vi "Movil SubVI.vi"(7 "Reset":bool, 8 "error in (no error)":errorcluster, 9 "Motor Izquierda":dbl(slide) scale=-100.0..100.0, 10 "Motor Derecha":dbl(slide) scale=-100.0..100.0, 11 "Ref Plano":refnum<vi>) -> (0 "error out":errorcluster, 1 "Distancia":dbl, 2 "Angulo":dbl, 3 "Plano de trabajo":picture, 5 "Button Down":bool)   [LabVIEW 2017]
uses:
  <vilib>/picture/picture.llb/imagedata.ctl
panel:
  out "new picture":picture
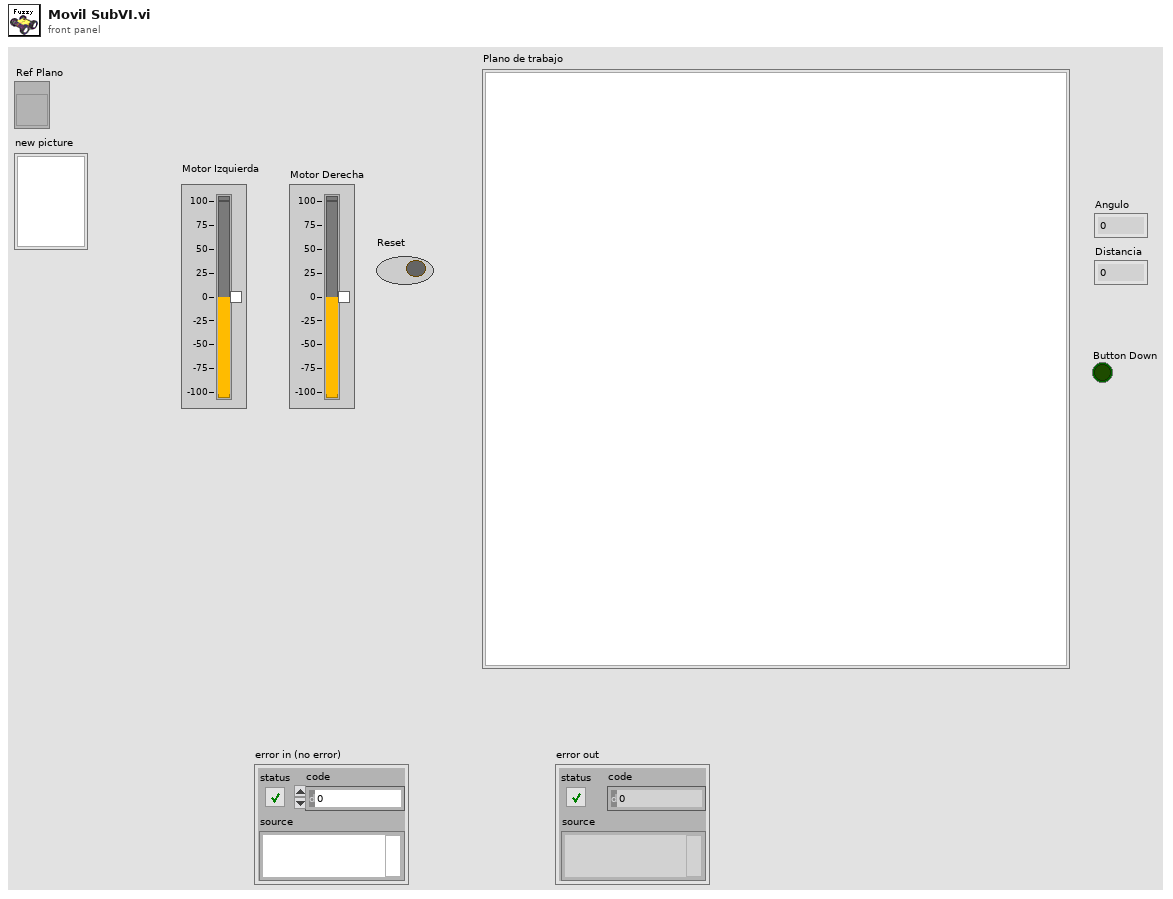
[diagram p1: front panel]
types:
  T1 = typedef "imagedata.ctl" = cluster{"image type":i32, "image depth":i32, "image":u8[], "mask":u8[], "colors":u32[], "Rectangle":cluster{"left":i16, "top":i16, "right":i16, "bottom":i16}}
  T2 = typedef "LVMouseTypeDef.ctl" = cluster{"Mouse Position":cluster{"X":i32, "Y":i32}, "Mouse Modifiers":cluster{"Button Down":bool, "Shift Mod":bool, "Menu Mod":bool, "Option Mod":bool}}
  T3 = cluster{"Button Down":bool, "Shift Mod":bool, "Menu Mod":bool, "Option Mod":bool}
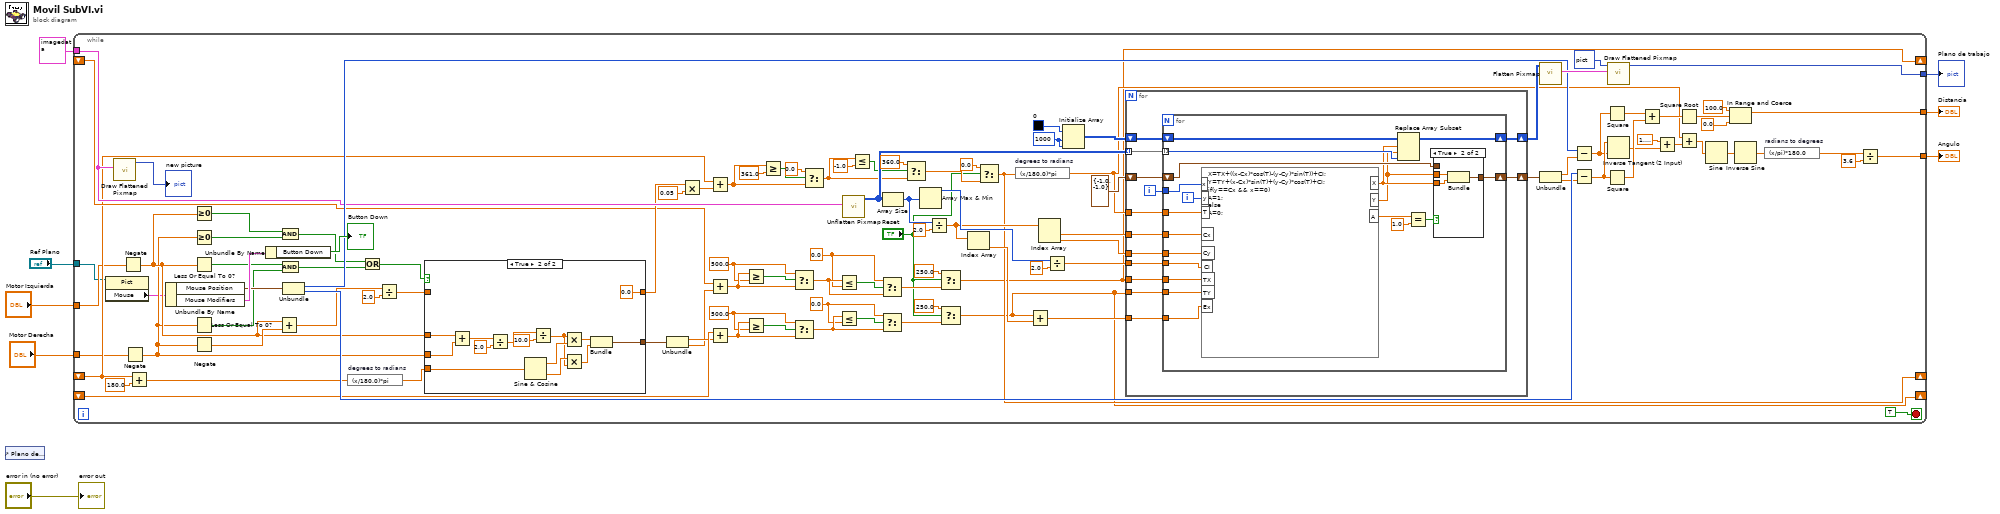
[diagram p0: block diagram]
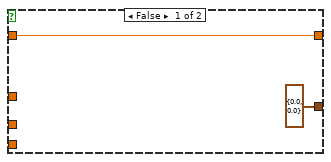
[diagram p2: hidden frame]
diagram:
  n1 = control-ref of="Plano de trabajo"() -> ()  [unwired: 1 out]
  n2 = while {
    shift-right: [w64] -> _
    shift-left: _ -> [w27]
    tunnel: T1 {"image type"=0, "image depth"=24, "image"=array[11970 elements], "mask"=[], "colors"=[], "Rectangle"={"left"=0, "top"=0, "right"=57, "bottom"=70}} ("image data") -> [w65]
    shift-right: [w24] -> _
    shift-left: _ -> [w38]
    shift-right: [w23] -> _
    shift-left: _ -> [w37]
    tunnel: "Motor Izquierda" -> [w17]
    tunnel: "Motor Derecha" -> [w16]
    tunnel: [w15] -> w5
    tunnel: [w14] -> w4
    tunnel: "Ref Plano" -> [w10]
    tunnel: [w9] -> w3
    stop <- TRUE stop-if-true
    w32 = 0.0 ("y")
    w34 = 500.0 ("y")
    w33 = 0.0 ("y")
    w35 = 500.0 ("y")
    w105 = 1000 ("dimension size")
    n3 = property class="Pict"(reference=w10) -> ("Mouse"=w11:T2)  [unwired: 1 in, 2 out]
    n4 = call <vilib>:"Draw Flattened Pixmap.vi"("image data"=w65) -> ("new picture"=→"new picture":picture)  [unwired: 8 in]
    n5 = Negate(x=w17) -> (-x=w13:dbl)
    n6 = Negate(x=w16) -> (-x=w12:dbl)
    n7 = Add(x=w27, y=180.0) -> (x+y=w25:dbl)
    n8 = Unbundle By Name(w11) -> ("Mouse Position"=w94:cluster{"X":i32, "Y":i32}, "Mouse Modifiers"=w104:T3)
    n9 = Greater Or Equal To 0?(x=w13) -> (x >= 0?=w59:bool)
    n10 = Greater Or Equal To 0?(x=w12) -> (x >= 0?=w58:bool)
    n11 = Less Or Equal To 0?(x=w13) -> (x <= 0?=w57:bool)
    n12 = Less Or Equal To 0?(x=w12) -> (x <= 0?=w56:bool)
    n13 = Negate(x=w12) -> (-x=w62:dbl)
    n14 = Unbundle By Name(w104) -> ("Button Down"=→"Button Down":bool)
    n15 = Add(x=w13, y=w62) -> (x+y=w61:dbl)
    n16 = And(x=w59, y=w58) -> (x .and. y?=w55:bool)
    n17 = And(x=w57, y=w56) -> (x .and. y?=w54:bool)
    n18 = Unbundle(w94) -> ("X"=w88:i32, "Y"=w90:i32)
    n19 = expression code="(x/180.0)*pi" "degrees to radians"(w25) -> (w31:dbl)
    n20 = Or(x=w55, y=w54) -> (x .or. y?=w53:bool)
    n21 = Divide(x=w61, y=2.0) -> (x/y=w52:dbl)
    n22 = case shown="True" w53 {
      tunnel: w52 -> [w118 _]
      tunnel: [w118 0.0] -> w51
      tunnel: w13 -> [_ w131]
      tunnel: w12 -> [_ w130]
      tunnel: w31 -> [_ w125]
      tunnel: [cluster{dbl, dbl} {0.0, 0.0} w119] -> w30
      frame False {
      }
      frame True {
        n23 = Add(x=w131, y=w130) -> (x+y=w129:dbl)
        n24 = Divide(x=w129, y=2.0) -> (x/y=w127:dbl)
        n25 = Sine & Cosine(0:w125) -> (1:w123:dbl, 2:w124:dbl)
        n26 = Divide(x=w127, y=10.0) -> (x/y=w122:dbl)
        n27 = Multiply(x=w122, y=w123) -> (x*y=w121:dbl)
        n28 = Multiply(x=w124, y=w122) -> (x*y=w120:dbl)
        n29 = Bundle(w121, w120) -> (w119:cluster{dbl, dbl})  [unwired: 1 in]
      }
    }
    n30 = Unbundle(w30) -> (w29:dbl, w28:dbl)
    n31 = Multiply(x=w51, y=0.05) -> (x*y=w69:dbl)
    n32 = Add(x=w27, y=w69) -> (x+y=w73:dbl)
    n33 = Add(x=w37, y=w28) -> (x+y=w43:dbl)
    n34 = Add(x=w38, y=w29) -> (x+y=w46:dbl)
    n35 = Greater Or Equal?(x=w43, y=w34) -> (x >= y?=w44:bool)
    n36 = Greater Or Equal?(x=w46, y=w35) -> (x >= y?=w45:bool)
    n37 = Greater Or Equal?(x=w73, y=361.0) -> (x >= y?=w75:bool)
    n38 = Select(t=w34, s=w44, f=w43) -> (s? t:f=w39:dbl)
    n39 = Select(t=w35, s=w45, f=w46) -> (s? t:f=w50:dbl)
    n40 = Select(t=0.0, s=w75, f=w73) -> (s? t:f=w66:dbl)
    n41 = Less Or Equal?(x=w39, y=w32) -> (x <= y?=w42:bool)
    n42 = Less Or Equal?(x=w50, y=w33) -> (x <= y?=w47:bool)
    n43 = call <vilib>:"Unflatten Pixmap.vi"("image data"=w65) -> ("24-bit pixmap"=w115:u32[][])  [unwired: 4 in, 6 out]
    n44 = Less Or Equal?(x=w66, y=-1.0) -> (x <= y?=w71:bool)
    n45 = Select(t=w32, s=w42, f=w39) -> (s? t:f=w40:dbl)
    n46 = Select(t=w33, s=w47, f=w50) -> (s? t:f=w49:dbl)
    n47 = Array Size(array=w115) -> (size(s)=w111:i32[])
    n48 = Select(t=360.0, s=w71, f=w66) -> (s? t:f=w67:dbl)
    n49 = Array Max & Min(array=w111) -> (max value=w109:i32)  [unwired: 3 out]
    n50 = Divide(x=w111, y=2.0) -> (x/y=w102:dbl[])
    n51 = Select(t=250.0, s="Reset", f=w40) -> (s? t:f=w23:dbl)
    n52 = Select(t=250.0, s="Reset", f=w49) -> (s? t:f=w24:dbl)
    n53 = Index Array(array=w102) -> (element=w101:dbl)  [unwired: 1 in]
    n54 = Select(t=0.0, s="Reset", f=w67) -> (s? t:f=w64:dbl)
    n55 = expression code="(x/180.0)*pi" "degrees to radians"(w64) -> (w82:dbl)
    n56 = Add(x=w24, y=w101) -> (x+y=w97:dbl)
    n57 = Index Array(array=w102) -> (element #1=w100:dbl, element #2=w99:dbl)  [unwired: 2 in]
    n58 = Divide(x=w109, y=2.0) -> (x/y=w98:dbl)
    n59 = Initialize Array(u32 0, w105, w105) -> (w108:u32[][])
    n60 = for {
      shift-right: [w141] -> w114
      shift-left: w108 -> [w145]
      tunnel: w82 -> [w143]
      tunnel: w115 -> [w142] mode=indexing
      tunnel: w100 -> [w140]
      tunnel: w99 -> [w139]
      tunnel: w98 -> [w138]
      tunnel: w23 -> [w137]
      tunnel: w24 -> [w136]
      tunnel: w97 -> [w135]
      shift-right: [w133] -> w95
      shift-left: cluster{dbl, dbl} {-1.0, -1.0} -> [w134]
      i -> [w144]
      n61 = for {
        shift-right: [w161] -> w141
        shift-left: w145 -> [w163]
        tunnel: w144 -> [w153]
        tunnel: w143 -> [w164]
        tunnel: w142 -> [w162] mode=indexing
        tunnel: w140 -> [w160]
        tunnel: w139 -> [w159]
        tunnel: w138 -> [w158]
        tunnel: w137 -> [w150]
        tunnel: w136 -> [w152]
        tunnel: w135 -> [w149]
        shift-right: [w154] -> w133
        shift-left: w134 -> [w157]
        i -> [w151]
        n62 = formula code="X=TX+((x-Cx)*cos(T)-(y-Cy)*sin(T))+CI;\nY=TY+(x-Cx)*sin(T)+(y-Cy)*cos(T)+CI;\nif(y==Cx && x==0)\nA=1;\nelse\nA=0;"("x"=w153, "y"=w151, "T"=w164, "Cx"=w160, "Cy"=w159, "CI"=w158, "TX"=w150, "TY"=w152, "Ex"=w149) -> ("X"=w156:dbl, "Y"=w155:dbl, "A"=w148:dbl)
        n63 = Replace Array Subset(array=w163, new element=w162, index (row)=w156, index (col)=w155) -> (w161:u32[][])
        n64 = Equal?(x=w148, y=1.0) -> (x = y?=w146:bool)
        n65 = case shown="True" w146 {
          tunnel: w157 -> [w165 _]
          tunnel: w156 -> [_ w166]
          tunnel: w155 -> [_ w167]
          tunnel: [w165 w168] -> w154
          frame False {
          }
          frame True {
            n66 = Bundle("Y"=w167, "X"=w166) -> (w168:cluster{"Y":dbl, "X":dbl})  [unwired: 1 in]
          }
        }
      }
    }
    n67 = call <vilib>:"Flatten Pixmap.vi"("24-bit pixmap"=w114) -> ("image data"=w106:T1)  [unwired: 10 in]
    n68 = Unbundle(w95) -> (w87:dbl, w89:dbl)
    n69 = Subtract(x=w88, y=w87) -> (x-y=w85:dbl)
    n70 = Subtract(x=w90, y=w89) -> (x-y=w86:dbl)
    n71 = Square(x=w85) -> (x^2=w92:dbl)
    n72 = Square(x=w86) -> (x^2=w93:dbl)
    n73 = call <vilib>:"Draw Flattened Pixmap.vi"("image data"=w106, "picture"=picture data[5B]) -> ("new picture"=w9:picture)  [unwired: 7 in]
    n74 = Inverse Tangent (2 Input)(1:w85, 2:w86) -> (0:w80:dbl)
    n75 = Add(x=w92, y=w93) -> (x+y=w91:dbl)
    n76 = Add(x=1.5707963267948966, y=w80) -> (x+y=w84:dbl)
    n77 = Square Root(x=w91) -> (sqrt(x)=w20:dbl)
    n78 = Add(x=w82, y=w84) -> (x+y=w79:dbl)
    n79 = Sine(x=w79) -> (sin(x)=w83:dbl)
    n80 = In Range and Coerce(upper limit=100.0, x=w20, lower limit=0.0) -> (coerced(x)=w14:dbl)  [unwired: 1 out]
    n81 = Inverse Sine(1:w83) -> (0:w78:dbl)
    n82 = expression code="(x/pi)*180.0" "radians to degrees"(w78) -> (w22:dbl)
    n83 = Divide(x=w22, y=3.6) -> (x/y=w15:dbl)
  }
  "Angulo" <- w5
  "Distancia" <- w4
  "Plano de trabajo" <- w3
  "error out" <- "error in (no error)"
